vi "Register Search.vi"(8 "error in (no error)":errorcluster, 10 "Search":refnum<class "Search.lvclass">, 11 "BetterSearch in":refnum<class "BetterSearch.lvclass">) -> (0 "error out":errorcluster, 3 "BetterSearch out":refnum<class "BetterSearch.lvclass">)   [LabVIEW 2020, in "Better Search.lvlib" / "BetterSearch.lvclass"]
uses:
  BetterSearch.lvclass
  Search/Search.lvclass
  BetterSearch.lvclass/BetterSearch.ctl
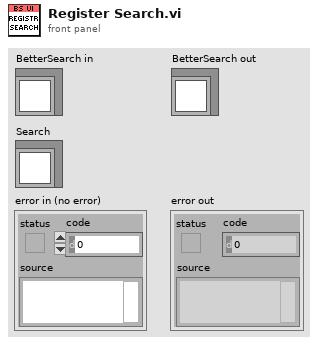
[diagram p1: front panel]
types:
  T1 = typedef "Better Search.lvlib/Search Params.ctl" = cluster{"Type":T2, "Type ID":string, "Text":string, "Scope":T3, "Targets":refnum<vi>[], "Scope Options":T4, "Typedef Path":path, "Member Graph Index":i32, "Member TypeID":string}
  T2 = typedef "Better Search.lvlib/Search Type.ctl" = enum16{"Generic", "Text", "Data Type", "VI", "Node"}
  T3 = typedef "Better Search.lvlib/Search Scope.ctl" = enum16{"Active Target", "Active Project", "Specific Targets", "Active VI", "Active Hierarchy"}
  T4 = typedef "Better Search.lvlib/Scope Options.ctl" = cluster{"Include Labels":bool, "Include Captions":bool, "Include Node Name":bool, "Member Access":bool, "Member Read":bool, "Member Write":bool, "Member Name":string, "String Value":bool, "Dependencies":bool, "vi.lib":bool, "user.lib":bool, "instr.lib":bool}
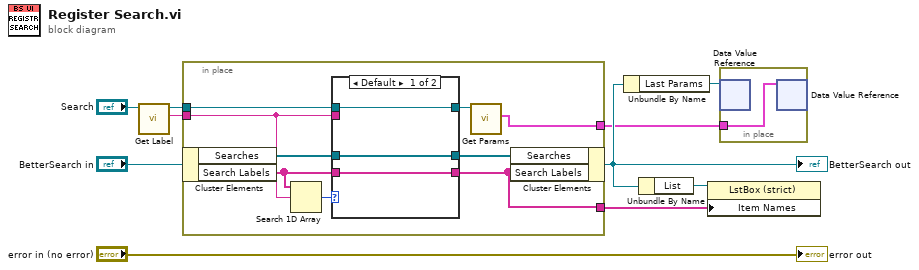
[diagram p0: block diagram]
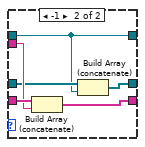
[diagram p2: hidden frame]
diagram:
  n1 = call "Get Label.vi"("Search in"="Search") -> ("Label"=w6:string, "Search out"=w7:refnum<class "Search.lvclass">)  [unwired: 8 in, 1 out]
  n2 = in-place {
    in-place-border: w7 -> [w16]
    in-place-border: w6 -> [w15]
    in-place-border: [w13] -> w4
    in-place-border: [w11] -> w1
    n3 = in-place-cluster #1("BetterSearch in") -> ("Searches"=w19:refnum<class "Search.lvclass">[], "Search Labels"=w17:string[])
    n4 = Search 1D Array(1D array=w17, element=w15) -> (index of element=w18:i32)  [unwired: 1 in]
    n5 = case shown="Default" w18 {
      tunnel: w19 -> [w21 w26]
      tunnel: w17 -> [w22 w28]
      tunnel: w16 -> [w20 w23]
      tunnel: w15 -> [_ w27]
      tunnel: [w22 w25] -> w13
      tunnel: [w21 w24] -> w14
      tunnel: [w20 w23] -> w12
      frame Default {
      }
      frame -1 {
        n6 = Build Array (concatenate)(w28, w27) -> (w25:string[])
        n7 = Build Array (concatenate)(w26, w23) -> (w24:refnum<class "Search.lvclass">[])
      }
    }
    n8 = call "Get Params.vi"("Search in"=w12) -> ("Params"=w11:T1)  [unwired: 8 in, 2 out]
    n9 = in-place-cluster #1("Searches"=w14, "Search Labels"=w13) -> (w2:refnum<class "BetterSearch.lvclass">)
  }
  "BetterSearch out" <- w2
  n10 = Unbundle By Name(w2) -> ("Last Params"=w3:refnum<data-value>)
  n11 = Unbundle By Name(w2) -> ("List"=w5:refnum<vi>)
  n12 = property class="LstBox (strict)"(reference=w5, "Item Names"=w4) -> ()  [unwired: 1 in, 2 out]
  n13 = in-place {
    in-place-border: w1 -> [w29]
    n14 = in-place-dvr #2(w3) -> ()  [unwired: 2 out]
    n15 = in-place-dvr #2(w29) -> ()  [unwired: 2 out]
  }
  "error out" <- "error in (no error)"
